vi "Register Mouse Events.vi"(8 "error in (no error)":errorcluster, 11 "Picture in":refnum<vi>) -> (0 "error out":errorcluster, 1 "CB VIs":refnum<vi>[](array[refnum]), 2 "event callback refnum":refnum<k27>, 3 "Cluster":T1)   [LabVIEW 2015, in "LV Image Editor Framework.lvlib" / "Image Editor Handler.lvclass"]
uses:
  Image Editor Handler.lvclass
  <vilib>/Utility/miscctls.llb/LVPoint32TypeDef.ctl
  Callbacks/Handler UI Callbacks.lvlib
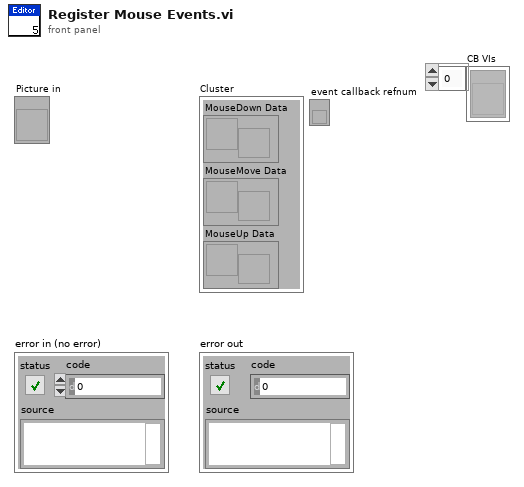
[diagram p1: front panel]
types:
  T1 = cluster{"MouseDown Data":refnum<user-event>, "MouseMove Data":refnum<user-event>, "MouseUp Data":refnum<user-event>}
  T2 = typedef "LVPoint32TypeDef.ctl" = cluster{"Horizontal":i32, "Vertical":i32}
  T3 = cluster{"Coords":T2, "Button":u16, "Mods":cluster{"Double Click":bool, "Menu Key":bool}, "PlatMods":cluster{"Shift":bool, "Ctrl":bool, "Alt":bool, "Cmd":bool, "Opt":bool}}
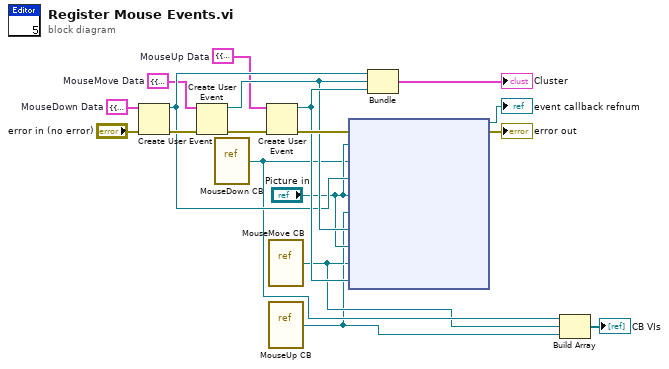
[diagram p0: block diagram]
diagram:
  w8 = T3 {"Coords"={"Horizontal"=0, "Vertical"=0}, "Button"=0, "Mods"={"Double Click"=FALSE, "Menu Key"=FALSE}, "PlatMods"={"Shift"=FALSE, "Ctrl"=FALSE, "Alt"=FALSE, "Cmd"=FALSE, "Opt"=FALSE}}  # MouseUp Data
  w7 = cluster{"Coords":T2} {"Coords"={"Horizontal"=0, "Vertical"=0}}  # MouseMove Data
  w6 = T3 {"Coords"={"Horizontal"=0, "Vertical"=0}, "Button"=0, "Mods"={"Double Click"=FALSE, "Menu Key"=FALSE}, "PlatMods"={"Shift"=FALSE, "Ctrl"=FALSE, "Alt"=FALSE, "Cmd"=FALSE, "Opt"=FALSE}}  # MouseDown Data
  n1 = Create User Event(user event datatype=w6, error in="error in (no error)") -> (user event=w10:refnum<user-event>, error out=w15:errorcluster)
  n2 = Create User Event(user event datatype=w7, error in=w15) -> (user event=w11:refnum<user-event>, error out=w16:errorcluster)
  n3 = vi-ref "MouseDown CB.vi"() -> ("vi reference"=w4:refnum<vi>)
  n4 = Create User Event(user event datatype=w8, error in=w16) -> (user event=w12:refnum<user-event>, error out=w17:errorcluster)
  n5 = vi-ref "MouseMove CB.vi"() -> ("vi reference"=w3:refnum<vi>)
  n6 = vi-ref "MouseUp CB.vi"() -> ("vi reference"=w2:refnum<vi>)
  n7 = node(w17, "Picture in", w4, w10, "Picture in", w3, w11, "Picture in", w2, w12) -> (→"event callback refnum":refnum<k27>, →"error out":errorcluster)  [unwired: 1 in]
  n8 = Bundle("MouseDown Data"=w10, "MouseMove Data"=w11, "MouseUp Data"=w12) -> (→"Cluster":T1)  [unwired: 1 in]
  n9 = Build Array(w4, w3, w2) -> (→"CB VIs":refnum<vi>[])
